vi "Washer_DSM_CMD.vi"(10 "Command":u8(ring)=2 items=["CMD_Entry_Command", "CMD_Load_Control", "RQST_Input_Status", "CMD_LED_Control", "RQST_Encoder_Position_Status", "RQST_A2D_Status", "RQST_Switch_States_Status", "CMD_Buzzer_Control", "CMD_Shift_to_Spin", "CMD_Shift_to_Agitate", "RQST_Mode_Shift_Complete_Status", "CMD_Control_Inverter", "CMD_Spin_Action", "CMD_Agitate_Action", "RQST_Total_Switch_Status", "RQST_Total_Encoder_Status", "CMD_Test_Eeprom", "RQST_Eeprom_Test_Status", "CMD_Power_Mode", "RQST_Error_Status", "RQST_Get_Version", "CMD_Set_Personality", "RQST_Get_Personality", "CMD_Serial_Number", "RQST_Serial_Number_Status", "CMD_Model_Number", "RQST_Model_Number_Status", "CMD_Enter_Boot_Loader", "CMD_Enable_Debug_Log"]) -> (1 "Info":string, 2 "CMD Byte":u8[](array[numeric])=[115, 0] format="%02x")   [LabVIEW 2016]
panel:
  in  "Commands":T1(array[cluster])=[{"CMD"="CMD_Entry_Command", "CMD Array"=[144], "Info"="[0]\n   - 0 = Exit EOL Test Mode\n   - 1 = Enter EOL Test Mode"}, {"CMD"="CMD_Load_Control", "CMD Array"=[50], "Info"="Refer to section 2.3.2.4 (Load Control Data)"}, {"CMD"="RQST_Input_Status", "CMD Array"=[51], "Info"="Refer to section 2.3.2.5 (Input Status)"}, {"CMD"="CMD_LED_Control", "CMD Array"=[147], "Info"="0-10] - LED States\n    Bit 0 - LED 0 (0 = Off, 1 = On)\n    Bit 1 - LED 1 (0 = Off, 1 = On)\n    ….\n    Bit 111 - LED 111 (0 = Off, 1 = On)\n[11-14] - LED States\n    SEG 0 (00 = Off, FF = On)\n    COLON (00 = Off, FF = On)\n    SEG 1(00 = Off, FF = On)\n    SEG 2(00 = Off, FF = On)"}, {"CMD"="RQST_Encoder_Position_Status", "CMD Array"=[148], "Info"="[0] - Encoder Position (0-15)"}, {"CMD"="RQST_A2D_Status", "CMD Array"=[98], "Info"="[0] - Requested Channel\n[1-2] - A2D Channel (MSB + LSB)"}, {"CMD"="RQST_Switch_States_Status", "CMD Array"=[149], "Info"="[0 - 3]\n  Bit 0 - Key 0 (1 = Released, 0 = Pressed)\n  Bit 1 - Key 1 (1 = Released, 0 = Pressed)\n  ….\n  Bit 31 - Key 31 (1 = Released, 0 = Pressed)"}, {"CMD"="CMD_Buzzer_Control", "CMD Array"=[150], "Info"="[0-1] - Buzzer frequency in Hz\n[2] - Buzzer Volume [0-100%]\n[3] - State (0 = Off, 1 = On)"}, {"CMD"="CMD_Shift_to_Spin", "CMD Array"=[128], "Info"="NA\n"}, {"CMD"="CMD_Shift_to_Agitate", "CMD Array"=[129], "Info"="NA"}, {"CMD"="RQST_Mode_Shift_Complete_Status", "CMD Array"=[132], "Info"="[0] - Mode Shift Complete Status (0 = Spin, 1 = Agitate)"}, {"CMD"="CMD_Control_Inverter", "CMD Array"=[80], "Info"="[0] - Command Type\n   0 - Spin\n   1 - Coast\n   2 - Brake\n   3 - OOB\n   4 - Load Size\n   5 - Dwell (used in ACM code for timing, never sent to Inverter)\n[1] - Direction(0 = CW, 1 = CCW)\n[2-3] - Target Speed (Basket RPM)\n[4-5] - Rate of Change"}, {"CMD"="CMD_Spin_Action", "CMD Array"=[120], "Info"="[0] = Profile Index"}, {"CMD"="CMD_Agitate_Action", "CMD Array"=[121], "Info"="[0] = Profile Index"}, {"CMD"="RQST_Total_Switch_Status", "CMD Array"=[134], "Info"="[0 - 3]\n  Bit 0 - Key 0 (0 = Pressed 1 = Not Pressed)\n  Bit 1 - Key 1 (0 = Pressed 1 = Not Pressed)\n  ….\n  Bit 31 - Key 31 (0 = Pressed 1 = Not Pressed)"}, {"CMD"="RQST_Total_Encoder_Status", "CMD Array"=[135], "Info"="[0 - 1]\n  Bit 0 - Position 0 (0 = Seen 1 = Unseen)\n  Bit 1 - Position 1 (0 = Seen 1 = Unseen\n  ….\n  Bit 15 - Position 15 (0 = Seen 1 = Unseen)"}, {"CMD"="CMD_Test_Eeprom", "CMD Array"=[151], "Info"="NA"}, {"CMD"="RQST_Eeprom_Test_Status", "CMD Array"=[152], "Info"="NA"}, {"CMD"="CMD_Power_Mode", "CMD Array"=[153], "Info"="[0] \n   - 0 = Normal Mode\n   - 1 = Low Power Mode"}, {"CMD"="RQST_Error_Status", "CMD Array"=[154], "Info"="[0-3] - Washer Errors\n[4-7] - Inverter Errors"}, {"CMD"="RQST_Get_Version", "CMD Array"=[1], "Info"="[0]-   Major_Version_Firmware\n[1]-   Minor_Version_Firmware\n[2]-   Major_Version_CriticalCode\n[3]-   Minor_Version_CriticalCode\n[4]-   Major_Version_ParametricData\n[5]-   Minor_Version_ParametricData\n[6]-   Major_Version_Inverter\n[7]-   Minor_Version_Inverter\n[8]-   Major_Version_InverterCritical\n[9]-   Minor_Version_InverterCritical\n[10]-   Major_Version_MachineControl\n[11]-   Minor_Version_MachineControl\n[12]-   Major_Version_MachineControlCritical\n[13]-   Minor_Version_MachineControlCritical\n[14]-   Major_Version_MachineControlEeprom\n[15]-   Minor_Version_MachineControlEeprom"}, {"CMD"="CMD_Set_Personality", "CMD Array"=[155], "Info"="[0] - Personality Number (0-15)"}, {"CMD"="RQST_Get_Personality", "CMD Array"=[157], "Info"="[0] - Personality Number (0-15)"}, {"CMD"="CMD_Serial_Number", "CMD Array"=[221], "Info"="[0] - 0x04 (Message ID)\n[1] - Completion Status\n   1 - Write Successful\n   2 - Not written, Data already present\n   3 - Not written, data too large\n   4 - write failed"}, {"CMD"="RQST_Serial_Number_Status", "CMD Array"=[221], "Info"="[0] - 0x03 (Message ID)\n[1] - Data Type\n   1 = Model Number\n    2 = Serial Number\n[2] - Length (1-24)\n[3-27] - Data  (ascii characters for Serial/Model"}, {"CMD"="CMD_Model_Number", "CMD Array"=[221], "Info"="[0] - 0x04  (Message ID)\n[1] -Data Type\n    1 = Model Number\n    2 = Serial Number\n[2] - Length of Data (1-24)\n[3-27] - Data (ascii characters for Serial/Model"}, {"CMD"="RQST_Model_Number_Status", "CMD Array"=[221], "Info"="[0] - 0x03 (Message ID)\n[1] - Data Type\n    1 = Model Number\n    2 = Serial Number"}, {"CMD"="CMD_Enter_Boot_Loader", "CMD Array"=[221], "Info"="[0] - 0x07"}, {"CMD"="CMD_Enable_Debug_Log", "CMD Array"=[115], "Info"="[0] - 1 = Enable, 0 = Disable"}] {"CMD Array" format="%.0x"}
  out "Data Array":string[][](array[string])=[["CMD_Eval_Mode_Entry_CC1", "0x70", "0x01"], ["CMD_Eval_Mode_Entry_CC2", "0x70", "0x02"], ["CMD_Eval_Mode_Continue", "0x71", "N/A"], ["CMD_Send_DIAG_Info", "0x72", "N/A"], ["CMD_Enable_Debug_Log ", "0x73", "0x01"], ["CMD_Disable_Debug_Log ", "0x73", "0x00"], ["CMD_Send_Log_Data", "0x74", "N/A"]]
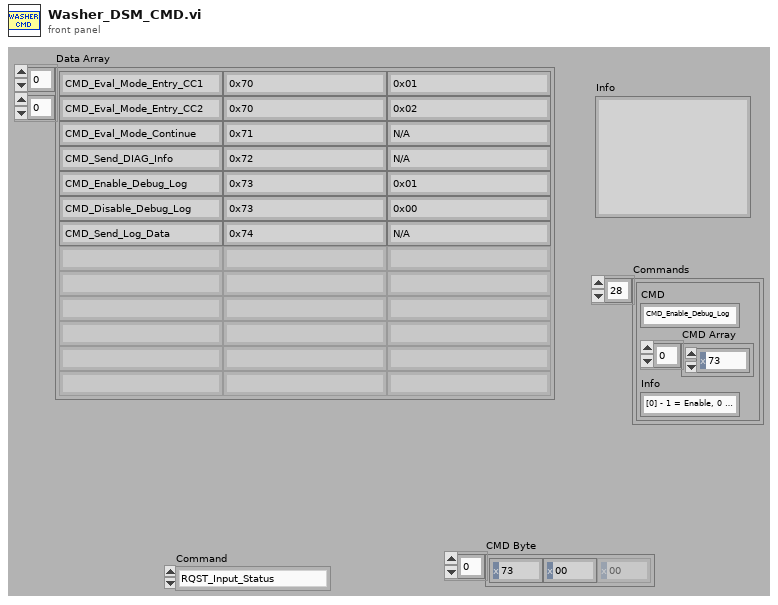
[diagram p1: front panel]
types:
  T1 = cluster{"CMD":string, "CMD Array":u8[], "Info":string}[]
  T2 = cluster{"CMD":string, "CMD Array":u8[], "Info":string}
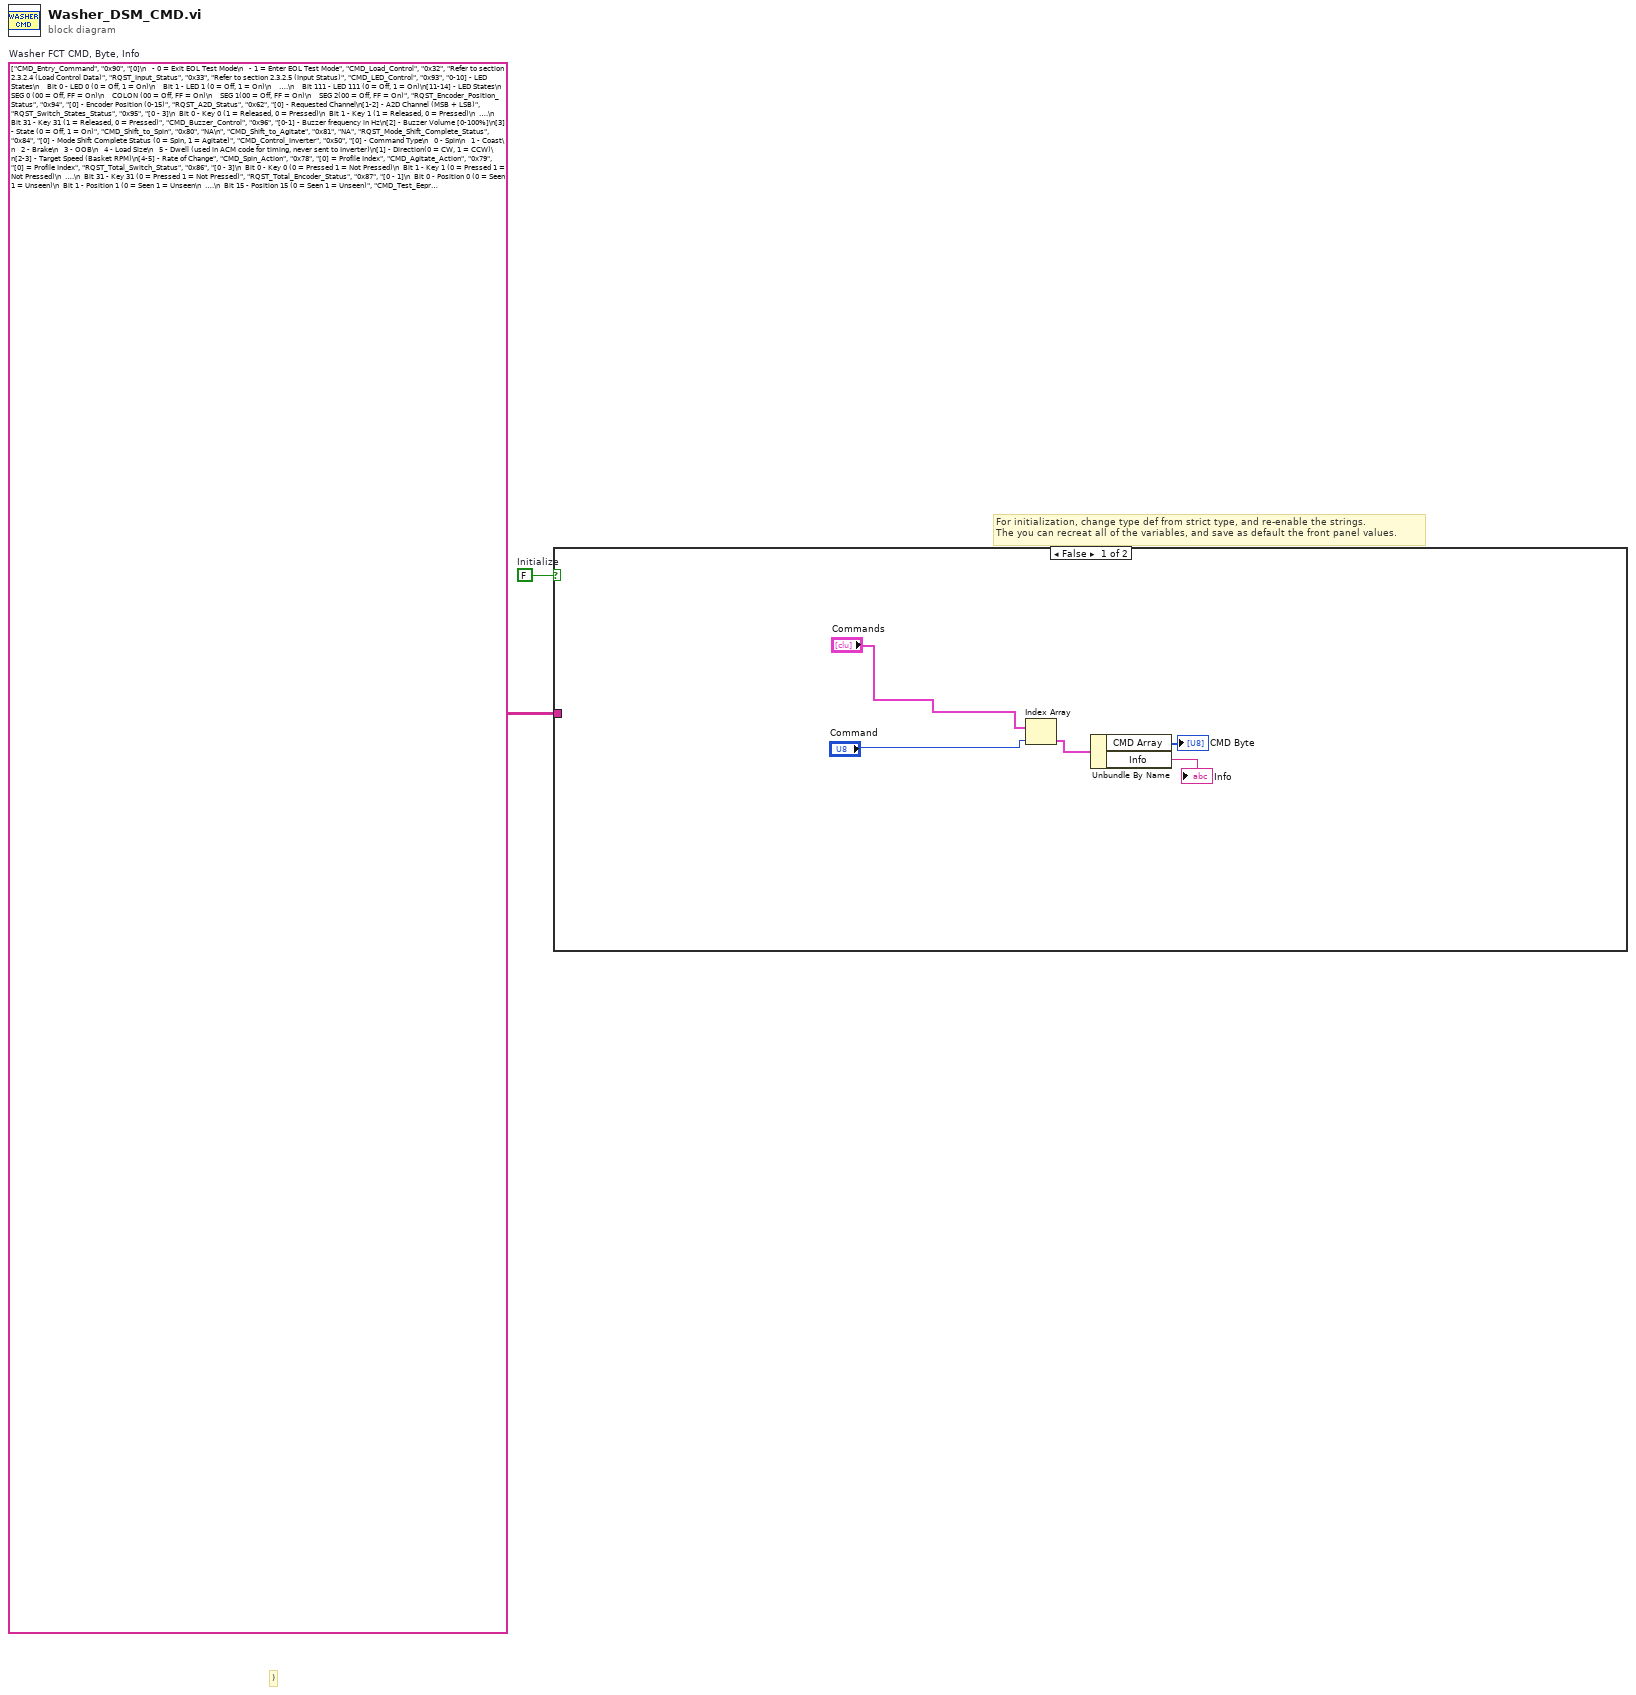
[diagram p0: block diagram]
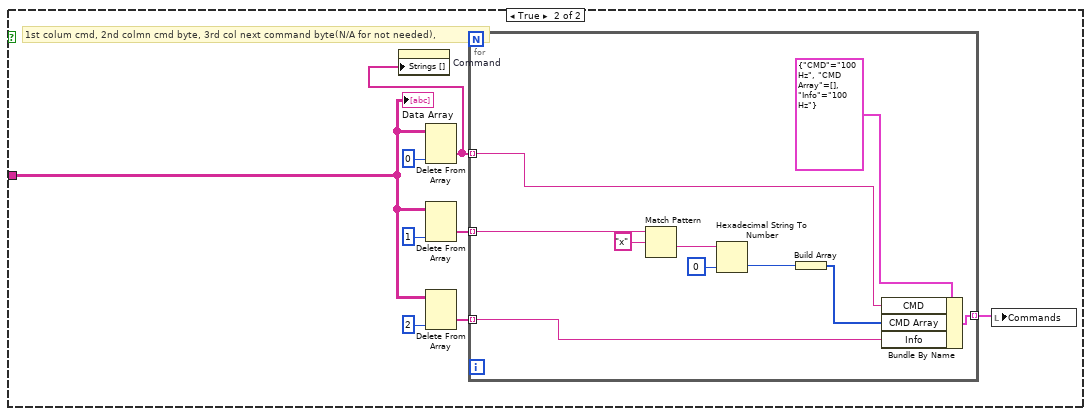
[diagram p2: hidden frame]
diagram:
  w1 = string[][] [["CMD_Entry_Command", "0x90", "[0]\n   - 0 = Exit EOL Test Mode\n   - 1 = Enter EOL Test Mode"], ["CMD_Load_Control", "0x32", "Refer to section 2.3.2.4 (Load Control Data)"], ["RQST_Input_Status", "0x33", "Refer to section 2.3.2.5 (Input Status)"], ["CMD_LED_Control", "0x93", "0-10] - LED States\n    Bit 0 - LED 0 (0 = Off, 1 = On)\n    Bit 1 - LED 1 (0 = Off, 1 = On)\n    ….\n    Bit 111 - LED 111 (0 = Off, 1 = On)\n[11-14] - LED States\n    SEG 0 (00 = Off, FF = On)\n    COLON (00 = Off, FF = On)\n    SEG 1(00 = Off, FF = On)\n    SEG 2(00 = Off, FF = On)"], ["RQST_Encoder_Position_Status", "0x94", "[0] - Encoder Position (0-15)"], ["RQST_A2D_Status", "0x62", "[0] - Requested Channel\n[1-2] - A2D Channel (MSB + LSB)"], ["RQST_Switch_States_Status", "0x95", "[0 - 3]\n  Bit 0 - Key 0 (1 = Released, 0 = Pressed)\n  Bit 1 - Key 1 (1 = Released, 0 = Pressed)\n  ….\n  Bit 31 - Key 31 (1 = Released, 0 = Pressed)"], ["CMD_Buzzer_Control", "0x96", "[0-1] - Buzzer frequency in Hz\n[2] - Buzzer Volume [0-100%]\n[3] - State (0 = Off, 1 = On)"], ["CMD_Shift_to_Spin", "0x80", "NA\n"], ["CMD_Shift_to_Agitate", "0x81", "NA"], ["RQST_Mode_Shift_Complete_Status", "0x84", "[0] - Mode Shift Complete Status (0 = Spin, 1 = Agitate)"], ["CMD_Control_Inverter", "0x50", "[0] - Command Type\n   0 - Spin\n   1 - Coast\n   2 - Brake\n   3 - OOB\n   4 - Load Size\n   5 - Dwell (used in ACM code for timing, never sent to Inverter)\n[1] - Direction(0 = CW, 1 = CCW)\n[2-3] - Target Speed (Basket RPM)\n[4-5] - Rate of Change"], ["CMD_Spin_Action", "0x78", "[0] = Profile Index"], ["CMD_Agitate_Action", "0x79", "[0] = Profile Index"], ["RQST_Total_Switch_Status", "0x86", "[0 - 3]\n  Bit 0 - Key 0 (0 = Pressed 1 = Not Pressed)\n  Bit 1 - Key 1 (0 = Pressed 1 = Not Pressed)\n  ….\n  Bit 31 - Key 31 (0 = Pressed 1 = Not Pressed)"], ["RQST_Total_Encoder_Status", "0x87", "[0 - 1]\n  Bit 0 - Position 0 (0 = Seen 1 = Unseen)\n  Bit 1 - Position 1 (0 = Seen 1 = Unseen\n  ….\n  Bit 15 - Position 15 (0 = Seen 1 = Unseen)"], ["CMD_Test_Eeprom", "0x97", "NA"], ["RQST_Eeprom_Test_Status", "0x98", "NA"], ["CMD_Power_Mode", "0x99", "[0] \n   - 0 = Normal Mode\n   - 1 = Low Power Mode"], ["RQST_Error_Status", "0x9A", "[0-3] - Washer Errors\n[4-7] - Inverter Errors"], ["RQST_Get_Version", "0x01", "[0]-   Major_Version_Firmware\n[1]-   Minor_Version_Firmware\n[2]-   Major_Version_CriticalCode\n[3]-   Minor_Version_CriticalCode\n[4]-   Major_Version_ParametricData\n[5]-   Minor_Version_ParametricData\n[6]-   Major_Version_Inverter\n[7]-   Minor_Version_Inverter\n[8]-   Major_Version_InverterCritical\n[9]-   Minor_Version_InverterCritical\n[10]-   Major_Version_MachineControl\n[11]-   Minor_Version_MachineControl\n[12]-   Major_Version_MachineControlCritical\n[13]-   Minor_Version_MachineControlCritical\n[14]-   Major_Version_MachineControlEeprom\n[15]-   Minor_Version_MachineControlEeprom"], ["CMD_Set_Personality", "0x9B", "[0] - Personality Number (0-15)"], ["RQST_Get_Personality", "0x9D", "[0] - Personality Number (0-15)"], ["CMD_Serial_Number", "0xDD", "[0] - 0x04 (Message ID)\n[1] - Completion Status\n   1 - Write Successful\n   2 - Not written, Data already present\n   3 - Not written, data too large\n   4 - write failed"], ["RQST_Serial_Number_Status", "0xDD", "[0] - 0x03 (Message ID)\n[1] - Data Type\n   1 = Model Number\n    2 = Serial Number\n[2] - Length (1-24)\n[3-27] - Data  (ascii characters for Serial/Model"], ["CMD_Model_Number", "0xDD", "[0] - 0x04  (Message ID)\n[1] -Data Type\n    1 = Model Number\n    2 = Serial Number\n[2] - Length of Data (1-24)\n[3-27] - Data (ascii characters for Serial/Model"], ["RQST_Model_Number_Status", "0xDD", "[0] - 0x03 (Message ID)\n[1] - Data Type\n    1 = Model Number\n    2 = Serial Number"], ["CMD_Enter_Boot_Loader", "0xDD", "[0] - 0x07"], ["CMD_Enable_Debug_Log", "0x73", "[0] - 1 = Enable, 0 = Disable"]]  # Washer FCT CMD, Byte, Info
  w2 = FALSE  # Initialize
  # ")"
  # "For initialization, change type def from strict type, and re-enable the strings.\nThe you can recreat all of the variables, and save as default the front panel values."
  n1 = case shown="False" w2 {
    tunnel: w1 -> [_ w10]
    frame False {
      n2 = Index Array(array="Commands", index="Command") -> (element=w7:T2)
      n3 = Unbundle By Name(w7) -> ("CMD Array"=→"CMD Byte":u8[], "Info"=→"Info":string)
    }
    frame True {
      # "1st colum cmd, 2nd colmn cmd byte, 3rd col next command byte(N/A for not needed),"
      n4 = Delete From Array(array=w10, index (col)=0 ("disabled index (col)")) -> (deleted portion=w9:string[])  [unwired: 2 in, 1 out]
      n5 = property on="Command" class="Ring (strict)"("Strings []"=w9) -> ()  [unwired: 2 in, 2 out]
      n6 = Delete From Array(array=w10, index (col)=1 ("disabled index (col)")) -> (deleted portion=w13:string[])  [unwired: 2 in, 1 out]
      n7 = Delete From Array(array=w10, index (col)=2 ("disabled index (col)")) -> (deleted portion=w11:string[])  [unwired: 2 in, 1 out]
      n8 = for {
        tunnel: w9 -> [w24] mode=indexing
        tunnel: w13 -> [w23] mode=indexing
        tunnel: [w22] -> w8 mode=indexing
        tunnel: w11 -> [w16] mode=indexing
        n9 = Match Pattern(string=w23, regular expression="x") -> (after substring=w19:string)  [unwired: 1 in, 3 out]
        n10 = Hexadecimal String To Number(string=w19, default (0uL)=u8 0 ("default (0 U32)")) -> (number=w17:u8)  [unwired: 1 in, 1 out]
        n11 = Build Array(w17) -> (w21:u8[])
        n12 = Bundle By Name(cluster=T2 {"CMD"="100 Hz", "CMD Array"=[], "Info"="100 Hz"}, "CMD"=w24, "CMD Array"=w21, "Info"=w16) -> (w22:T2)
      }
      n13 = local write "Commands"(w8) -> ()
      "Data Array" <- w10
    }
  }
